vi "List Cluster Elements.vi"() -> ()   [LabVIEW 2013]
uses:
  Common Code/Dashboard UDP Packet.ctl
  Common Code/Dashboard UDP/Camera Controls.ctl
  Common Code/Dashboard UDP/Gyro Controls.ctl
  Common Code/Dashboard UDP/PID Params.ctl
  Common Code/Dashboard UDP/Encoder Controls.ctl
  Common Code/Dashboard UDP/Auto Shift Controls.ctl
  Common Code/Dashboard UDP/Auton Controls.ctl
  Common Code/Dashboard UDP/Shooter Controls.ctl
  Common Code/Dashboard UDP/Roller Controls.ctl
  Dashboard Code/Preferences/Named Control.ctl
panel:
  out "Named Controls":T1
  out "Result":bool
  out "Duplicates Count":i32
  out "Status":string
  out "Duplicates":string[](array[string])
  out "Elements Count":i32
  out "Elements":string[](array[string])
  in  "UDP Packet":T2
  # "Step 1 - Run this VI, with the"
  # "Line"
  # "Shooter"
  # "Down"
  # "Up"
  # "Feet"
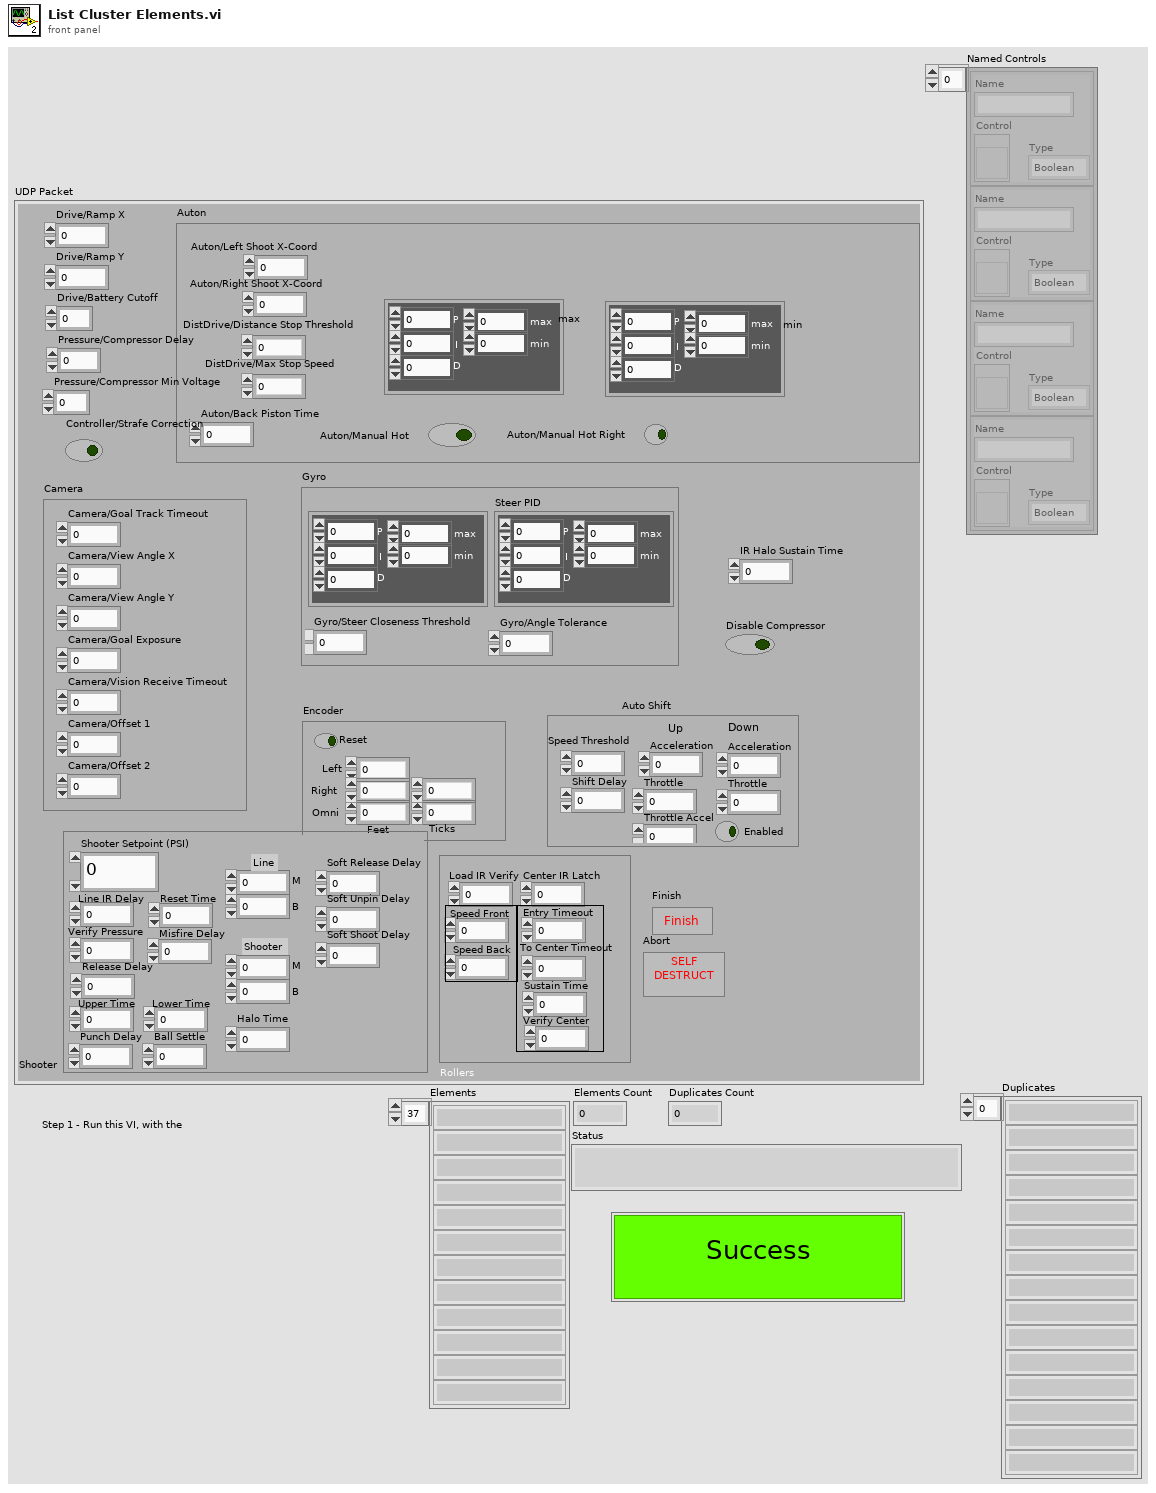
[diagram p1: front panel]
types:
  T1 = typedef "Named Control.ctl" = cluster{"Name":string, "Control":refnum<vi>, "Type":enum16{"Boolean", "Double"}}[]
  T2 = typedef "Dashboard UDP Packet.ctl" = cluster{"Camera":T3, "Gyro":T4, "Encoder":T6, "Auto Shift":T7, "Auton":T8, "Drive/Ramp X":dbl, "Drive/Ramp Y":dbl, "Drive/Battery Cutoff":dbl, "Pressure/Compressor Min Voltage":dbl, "Pressure/Compressor Delay":dbl, "Controller/Strafe Correction":bool, "Shooter":T9, "Rollers":T10, "Abort":bool, "Finish":bool, "IR Halo Sustain Time":dbl, "Disable Compressor":bool}
  T3 = typedef "Camera Controls.ctl" = cluster{"Camera/View Angle X":dbl, "Camera/Goal Track Timeout":dbl, "Camera/View Angle Y":dbl, "Camera/Goal Exposure":dbl, "Camera/Vision Receive Timeout":dbl, "Camera/Offset 1":dbl, "Camera/Offset 2":dbl}
  T4 = typedef "Gyro Controls.ctl" = cluster{"Gyro/Angle Tolerance":dbl, "Gyro/Steer Closeness Threshold":dbl, "Steer PID":T5, "Steer Close PID":T5}
  T5 = typedef "PID Params.ctl" = cluster{"max":dbl, "min":dbl, "P":dbl, "I":dbl, "D":dbl}
  T6 = typedef "Encoder Controls.ctl" = cluster{"Encoders/Reset":bool, "Encoders/Omni Constant":dbl, "Encoders/Omni Tick Constant":dbl, "Encoders/Left Constant":dbl, "Encoders/Right Constant":dbl, "Encoders/Right Tick Constant":dbl}
  T7 = typedef "Auto Shift Controls.ctl" = cluster{"AutoShift/Upshift Throttle Accel":dbl, "AutoShift/Speed Threshold":dbl, "AutoShift/Upshift Throttle":dbl, "AutoShift/Upshift Accel":dbl, "AutoShift/Downshift Accel":dbl, "AutoShift/Downshift Throttle":dbl, "AutoShift/Delay":dbl, "AutoShift/Enabled":bool}
  T8 = typedef "Auton Controls.ctl" = cluster{"Auton/Left Shoot X-Coord":dbl, "Auton/Right Shoot X-Coord":dbl, "DistDrive/Distance Stop Threshold":dbl, "DistDrive/Max Stop Speed":dbl, "Auton/Back Piston Time":dbl, "Auton/Manual Hot":bool, "Auton/Manual Hot Right":bool, "Default X PID":T5, "Default Y PID":T5}
  T9 = typedef "Shooter Controls.ctl" = cluster{"Shooter/Reset Time":dbl, "Shooter/Release Delay":dbl, "Shooter/Pressure Steady Time":dbl, "Shooter/Misfire Delay":dbl, "Shooter/Ball Settle Time":dbl, "Shooter/Line IR Delay":dbl, "Pressure/Upper PSI Time":dbl, "Pressure/Lower PSI Time":dbl, "Shooter/Punch Delay":dbl, "Shooter/Target Pressure":dbl, "Pressure/Line B":dbl, "Pressure/Line M":dbl, "Pressure/Shooter M":dbl, "Pressure/Shooter B":dbl, "Halo Time":dbl, "Soft Release Delay":dbl, "Soft Unpin Delay":dbl, "Soft Shoot Delay":dbl}
  T10 = typedef "Roller Controls.ctl" = cluster{"Roller/Load IRs Verify Time":dbl, "Roller/Center IR Latch Time":dbl, "Roller/Speed Front":dbl, "Roller/Speed Back":dbl, "Roller/Entry Timeout":dbl, "Roller/To Center Timeout":dbl, "Roller/Sustain Time":dbl, "Roller/Verify Center Time":dbl}
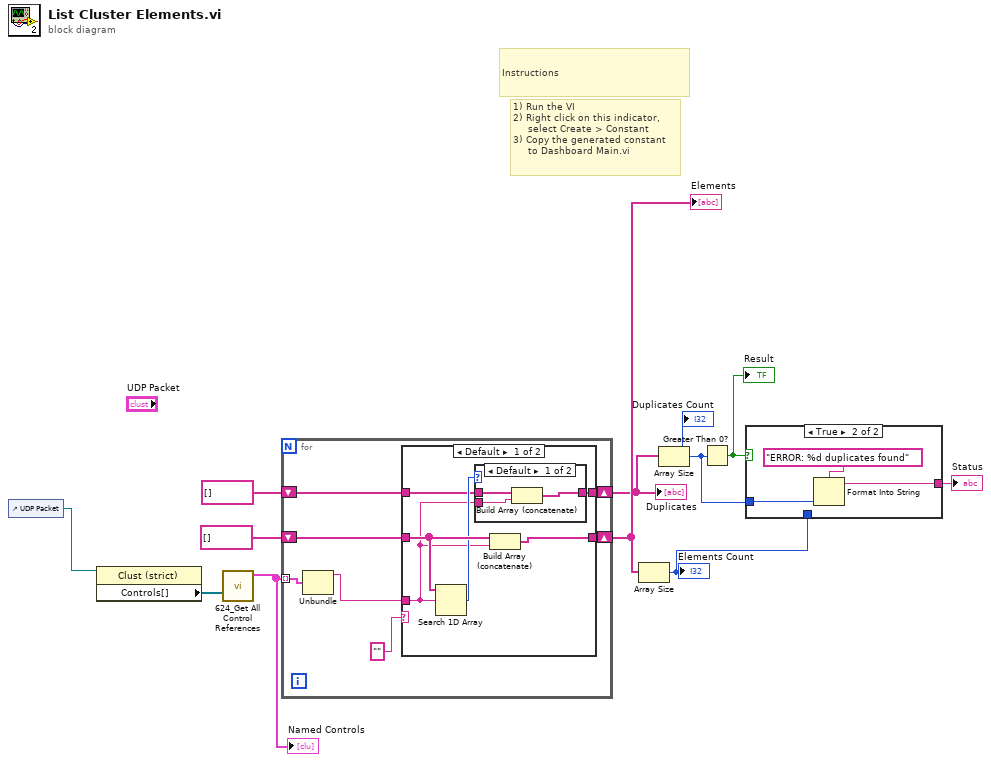
[diagram p0: block diagram]
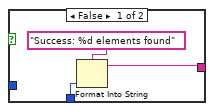
[diagram p2: hidden frame]
diagram:
  # "Instructions"
  # "1) Run the VI\n2) Right click on this indicator,\n     select Create > Constant\n3) Copy the generated constant\n     to Dashboard Main.vi"
  n1 = control-ref of="UDP Packet"() -> (w2:refnum<vi>)
  n2 = property class="Clust (strict)"(reference=w2) -> ("Controls[]"=w11:refnum<vi>[])  [unwired: 1 in, 2 out]
  n3 = call "624_Get All Control References.vi"("Controls[] in"=w11) -> ("Named Controls"=w1:T1)  [unwired: 8 in, 2 out]
  "Named Controls" <- w1
  n4 = for {
    shift-right: [w17] -> w9
    shift-left: string[] [] -> [w18]
    shift-right: [w15] -> w7
    shift-left: string[] [] -> [w16]
    tunnel: w1 -> [w12] mode=indexing
    n5 = Unbundle(w12) -> ("Name"=w13:string)  [unwired: 2 out]
    n6 = case shown="Default" "" {
      tunnel: w18 -> [w23 w30]
      tunnel: w13 -> [w20 _]
      tunnel: [w24 w30] -> w17
      tunnel: w16 -> [w21 w29]
      tunnel: [w19 w29] -> w15
      frame Default {
        n7 = Search 1D Array(1D array=w23, element=w20) -> (index of element=w22:i32)  [unwired: 1 in]
        n8 = case shown="Default" w22 {
          tunnel: w21 -> [w27 w28]
          tunnel: w20 -> [w26 _]
          tunnel: [w25 w28] -> w19
          frame Default {
            n9 = Build Array (concatenate)(w27, w26) -> (w25:string[])
          }
          frame -1 {
          }
        }
        n10 = Build Array (concatenate)(w23, w20) -> (w24:string[])
      }
      frame "Cluster" {
        # "Ignore Clusters"
      }
    }
  }
  "Elements" <- w9
  "Duplicates" <- w7
  n11 = Array Size(array=w9) -> (size(s)=w6:i32)
  "Elements Count" <- w6
  n12 = Array Size(array=w7) -> (size(s)=w4:i32)
  "Duplicates Count" <- w4
  n13 = Greater Than 0?(x=w4) -> (x > 0?=w3:bool)
  "Result" <- w3
  n14 = case shown="True" w3 {
    tunnel: [w31 w35] -> w5
    tunnel: w6 -> [w33 _]
    tunnel: w4 -> [_ w34]
    frame False {
      n15 = Format Into String(format string="Success: %d elements found", w33) -> (resulting string=w31:string)  [unwired: 2 in, 1 out]
    }
    frame True {
      n16 = Format Into String(format string="ERROR: %d duplicates found", w34) -> (resulting string=w35:string)  [unwired: 2 in, 1 out]
    }
  }
  "Status" <- w5
